vi "SQL_table_users_nonadmin_select_table.vi"() -> (0 "error out":errorcluster, 2 "普通用户个数":i32, 3 "普通用户信息":string[][](table))   [LabVIEW 2014]
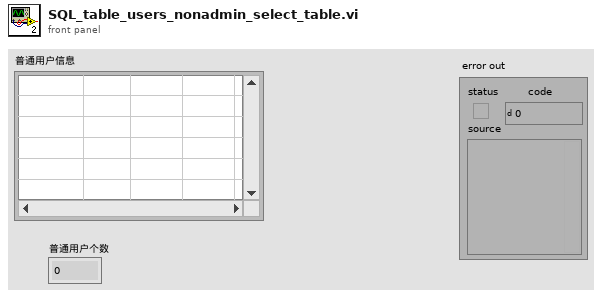
[diagram p1: front panel]
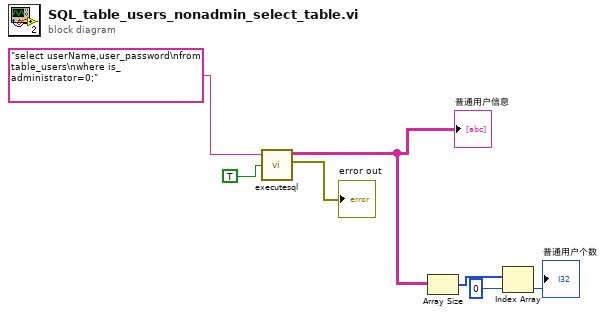
[diagram p0: block diagram]
diagram:
  n1 = call "executesql.vi"("Return Data (T)"=TRUE, "Command Text"="select userName,user_password\nfrom table_users\nwhere is_administrator=0;") -> ("error out"=→"error out":errorcluster, "Data"=w1:string[][])  [unwired: 5 in]
  "普通用户信息" <- w1
  n2 = Array Size(array=w1) -> (size(s)=w4:i32[])
  n3 = Index Array(array=w4, index=0) -> (element=→"普通用户个数":i32)
